vi "split image coordinates.vi"(7 "current array":picture[][](array[picture]), 8 "image select":picture) -> (2 "white Location out":T1, 3 "peice Location out":T1)   [LabVIEW 2014]
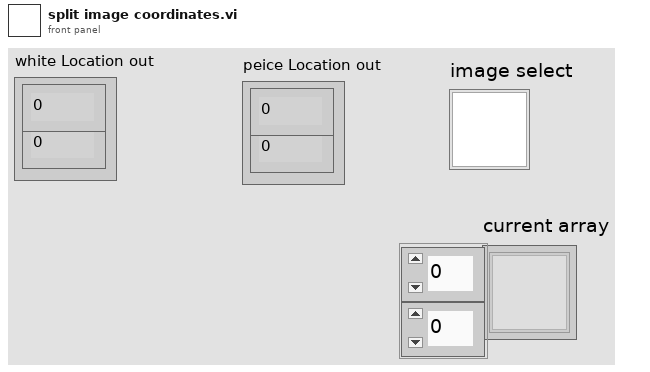
[diagram p1: front panel]
types:
  T1 = cluster{"Numeric Control":i32, "Numeric Control":i32}
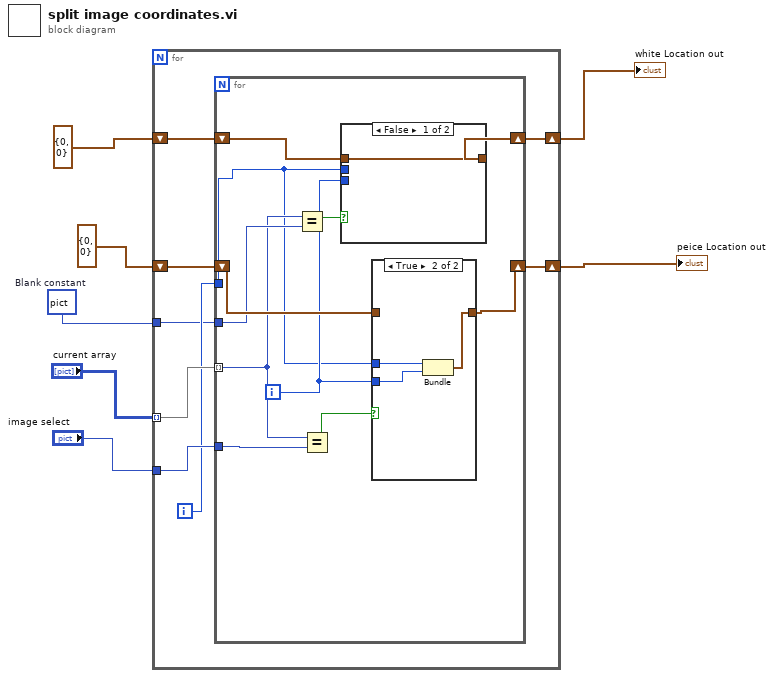
[diagram p0: block diagram]
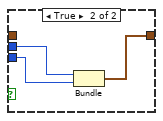
[diagram p2: hidden frame]
diagram:
  w3 = picture data[5B]  # Blank constant
  n1 = for {
    tunnel: "current array" -> [w15] mode=indexing
    tunnel: "image select" -> [w14]
    shift-right: [w12] -> w4
    shift-left: cluster{i32, i32} {0, 0} -> [w11]
    tunnel: w3 -> [w10]
    shift-right: [w9] -> w6
    shift-left: cluster{i32, i32} {0, 0} -> [w8]
    i -> [w13]
    n2 = for {
      tunnel: w15 -> [w21] mode=indexing
      tunnel: w14 -> [w26]
      tunnel: w13 -> [w18]
      shift-right: [w24] -> w12
      shift-left: w11 -> [w23]
      tunnel: w10 -> [w22]
      shift-right: [w17] -> w9
      shift-left: w8 -> [w16]
      i -> [w19]
      n3 = Equal?(x=w21, y=w22) -> (x = y?=w20:bool)
      n4 = Equal?(x=w21, y=w26) -> (x = y?=w25:bool)
      n5 = case shown="False" w20 {
        tunnel: w19 -> [_ w30]
        tunnel: w18 -> [_ w29]
        tunnel: [w27 w28] -> w17
        tunnel: w16 -> [w27 _]
        frame False {
        }
        frame True {
          n6 = Bundle(w29, w30) -> (w28:cluster{i32, i32})  [unwired: 1 in]
        }
      }
      n7 = case shown="True" w25 {
        tunnel: w18 -> [_ w33]
        tunnel: w19 -> [_ w32]
        tunnel: [w31 w34] -> w24
        tunnel: w23 -> [w31 _]
        frame False {
        }
        frame True {
          n8 = Bundle(w33, w32) -> (w34:cluster{i32, i32})  [unwired: 1 in]
        }
      }
    }
  }
  "white Location out" <- w6
  "peice Location out" <- w4
